vi "Simulate_kernal.vi"() -> (0 "error out":errorcluster)   [LabVIEW 2017]
uses:
  Globals/Meas_global.vi
  <vilib>/Analysis/NI_AALBase.lvlib
panel:
  out "Waveform Graph":dbl[][](graph)
  in  "Random?":bool
  in  "Average Value":dbl
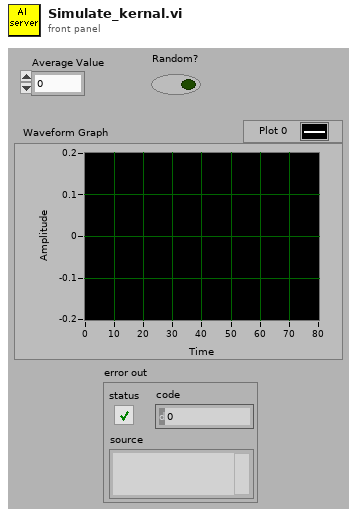
[diagram p1: front panel]
types:
  T1 = typedef "Analysis_info_cluster.ctl" = cluster{"Colour":u32, "Inst type":T2, "Inst name":string, "Symbol":string, "Code name":string, "Extra Info":string, "Inst Array":T3, "Extra Titles":string[], "Extra Values":string[], "U":dbl, "u^2":dbl, "u^3":dbl, "u^4":dbl, "Skew_u":dbl, "Kurt_u":dbl, "Sd Error in Mean":dbl, "% u'/U":dbl, "X":dbl, "Y":dbl, "Z":dbl, "Timescale integral Estimate":dbl, "Sd Error in Variance":dbl, "Calib File":path, "Calib Constants":dbl[], "Output Position":bool, "Full Stats":bool, "Av Sampling Rate":dbl, "Av No of Samples":dbl, "Total Meas Time (s)":dbl, "ADAM Ch Name":string, "Max value":dbl, "Min value":dbl, "Req Sample Rate Hz":dbl, "Sync Delay Time (s)":dbl, "Ch No":i16, "Device ID":string, "Use Latest Calib":bool, "Port":string}
  T2 = typedef "Inst_type.ctl" = enum16{"Propeller anemometer", "Raw voltage", "Pressure Transducer", "Pitot-static tube", "Preston tube", "Hot wire", "Cross wire 1", "Cross wire 2", "Generic Linear", "Generic Polynomial", "Generic BackPoly", "Fast FID", "Thermocouple", "Cold wire", "Pulsed Wire", "LDA Vel", "LDA Tran time", "LDA Arr time", "Microphone"}
  T3 = typedef "Instrument_Array.ctl" = enum16{"PWA", "LDA", "Analogue"}
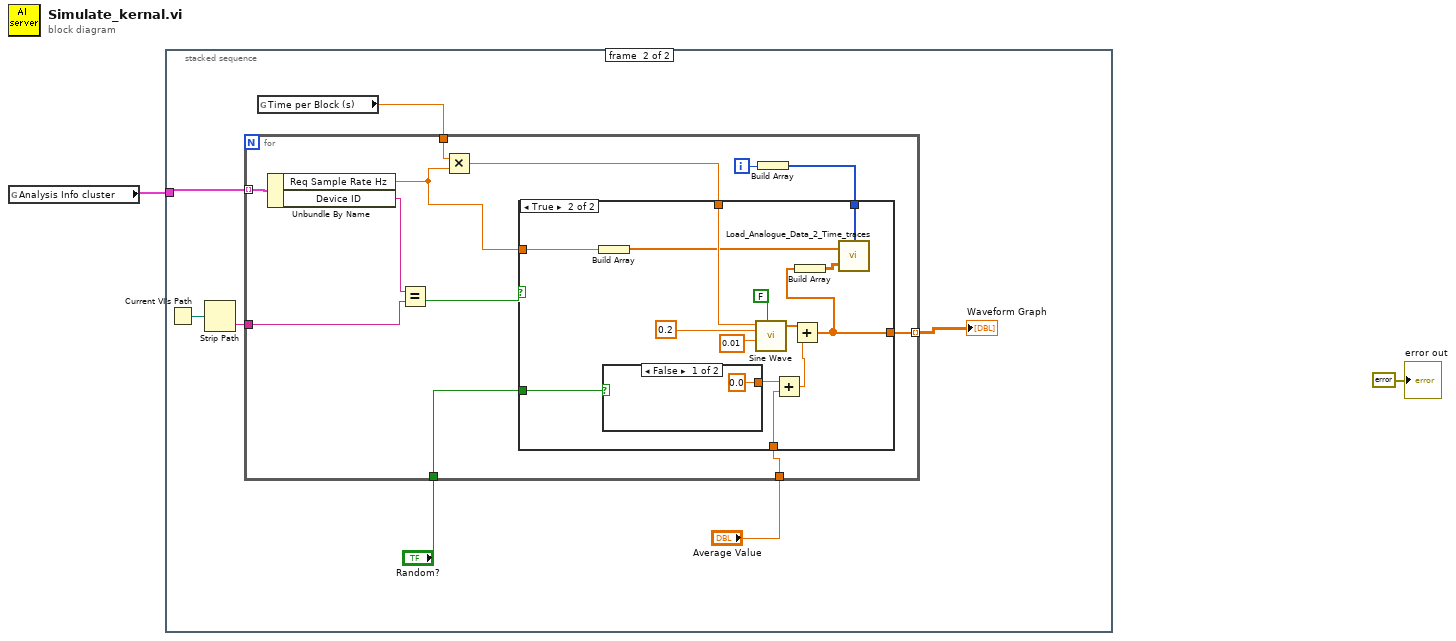
[diagram p0: block diagram]
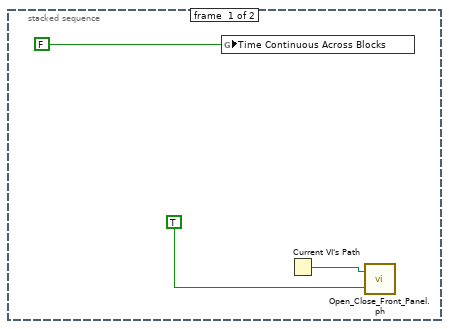
[diagram p2: hidden frame]
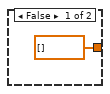
[diagram p3: hidden frame]
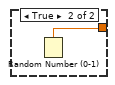
[diagram p4: hidden frame]
diagram:
  n1 = global read "Meas_global.vi" "Analysis Info cluster"() -> (w2:T1[])
  n2 = stacked-sequence {
    tunnel: w2 -> [_ w9]
    frame #0 {
      n3 = global write "Meas_global.vi" "Time Continuous Across Blocks"(FALSE ("Time Continuous across Blocks")) -> ()
      n4 = Current VI's Path() -> (path=w5:path)
      n5 = call "Open_Close_Front_Panel.ph.vi"("Front Panel Window:Open"=TRUE, "VI path"=w5) -> ()  [unwired: 2 out]
    }
    frame #1 {
      n6 = Current VI's Path() -> (path=w7:path)
      n7 = Strip Path(path=w7) -> (name=w6:string)  [unwired: 1 out]
      n8 = global read "Meas_global.vi" "Time per Block (s)"() -> (w8:dbl)
      n9 = for {
        tunnel: [w19] -> w10 mode=indexing
        tunnel: "Random?" -> [w24]
        tunnel: "Average Value" -> [w23]
        tunnel: w9 -> [w22] mode=indexing
        tunnel: w8 -> [w21]
        tunnel: w6 -> [w17]
        i -> [w15]
        n10 = Unbundle By Name(w22) -> ("Req Sample Rate Hz"=w13:dbl, "Device ID"=w18:string)
        n11 = Equal?(x=w18, y=w17) -> (x = y?=w16:bool)
        n12 = Multiply(x=w21, y=w13) -> (x*y=w20:dbl)
        n13 = Build Array(w15) -> (w14:i32[])
        n14 = case shown="True" w16 {
          tunnel: w24 -> [_ w36]
          tunnel: w23 -> [_ w33]
          tunnel: w20 -> [_ w31]
          tunnel: [dbl[] [] w27] -> w19
          tunnel: w14 -> [_ w30]
          tunnel: w13 -> [_ w29]
          frame False {
          }
          frame True {
            n15 = Build Array(w29) -> (w28:dbl[])
            n16 = case shown="False" w36 {
              tunnel: [0.0 ("number: 0 to 1") w41] -> w35
              frame False {
              }
              frame True {
                n17 = Random Number (0-1)() -> (number: 0 to 1=w41:dbl)
              }
            }
            n18 = call <vilib>:"Sine Wave.vi"("samples"=w31, "amplitude"=0.2, "frequency"=0.01 ("f"), "reset phase"=FALSE) -> ("sine wave"=w39:dbl[])  [unwired: 1 in, 2 out]
            n19 = Add(x=w35, y=w33) -> (x+y=w34:dbl)
            n20 = Add(x=w39, y=w34) -> (x+y=w27:dbl[])
            n21 = Build Array(w27) -> (w26:dbl[][])
            n22 = call "Load_Analogue_Data_2_Time_traces.vi"("Index"=w30, "Voltage Array"=w26, "Sampling Rate (Hz)"=w28) -> ()  [unwired: 1 in]
          }
        }
      }
      "Waveform Graph" <- w10
    }
  }
  "error out" <- errorcluster {"status"=FALSE, "code"=0, "source"=""} ("error out")
